vi "Funnel Edit.vi"() -> ()   [LabVIEW 2013]
uses:
  Global Variables.vi
panel:
  in  "Index":i32=8
  in  "Direction":u16(ring) items=["Forward", "Backward"]
  in  "Enabled":bool=TRUE
  in  "Voltage Schedule":u16(ring) items=["Constant", "Ramp", "Fn. Generator", "Formula"]
  in  "Apply to All":bool
  in  "Smooth Segments":dbl=12.0
  in  "Speed Schedule":u16(ring) items=["Constant", "Ramp", "Fn. Generator", "Formula"]
  in  "Speed (µm/s)":dbl=8.0 min=1e-09
  in  "Voltage (V)":dbl=8.0
  in  "Speed Settings":bool
  in  "Voltage Settings":bool
  in  "Bottom Segs.":dbl=0.1
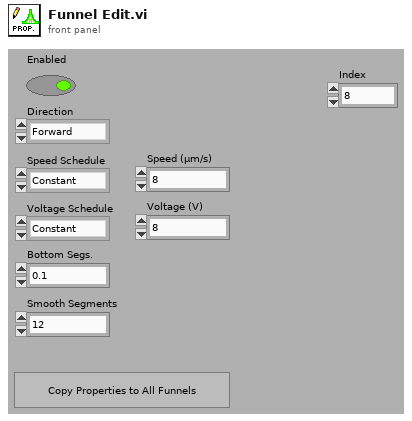
[diagram p1: front panel]
types:
  T1 = enum32{"invalid app kind", "Development System", "Run Time System", "Student Edition", "Embedded LabVIEW", "Evaluation", "Custom"}
  T2 = enum32{"Invalid", "Standard", "Closed", "Hidden", "Minimized", "Maximized"}
  T3 = cluster{"Enabled":bool, "Direction":u16, "Smooth Segments":dbl, "Bottom Segs.":dbl, "Speed (µm/s)":cluster{"Schedule":u16, "Value":dbl, "Start Value":dbl, "End Value":dbl, "Min Value":dbl, "Max Value":dbl, "Duty Cycle (%)":dbl, "Signal Type":u16, "Cycle Number":dbl, "Phase (degrees)":dbl}, "Voltage (V)":cluster{"Schedule":u16, "Value":dbl, "Start Value":dbl, "End Value":dbl, "Min Value":dbl, "Max Value":dbl, "Duty Cycle (%)":dbl, "Signal Type":u16, "Cycle Number":dbl, "Phase (degrees)":dbl}}[]
  T4 = cluster{"Enabled":bool, "Direction":u16, "Smooth Segments":dbl, "Bottom Segs.":dbl, "Speed (µm/s)":cluster{"Schedule":u16, "Value":dbl, "Start Value":dbl, "End Value":dbl, "Min Value":dbl, "Max Value":dbl, "Duty Cycle (%)":dbl, "Signal Type":u16, "Cycle Number":dbl, "Phase (degrees)":dbl}, "Voltage (V)":cluster{"Schedule":u16, "Value":dbl, "Start Value":dbl, "End Value":dbl, "Min Value":dbl, "Max Value":dbl, "Duty Cycle (%)":dbl, "Signal Type":u16, "Cycle Number":dbl, "Phase (degrees)":dbl}}
  T5 = cluster{"Schedule":u16, "Value":dbl, "Start Value":dbl, "End Value":dbl, "Min Value":dbl, "Max Value":dbl, "Duty Cycle (%)":dbl, "Signal Type":u16, "Cycle Number":dbl, "Phase (degrees)":dbl}
  T6 = cluster{"Schedule":u16, "Value":dbl, "Start Value":dbl, "End Value":dbl, "Min Value":dbl, "Max Value":dbl, "Duty Cycle (%)":dbl, "Speed Signal Type":u16, "Cycle Number":dbl, "Phase (degrees)":dbl}
  T7 = cluster{"Core":cluster{"Current VI Reference":refnum<vi>, "Close Panel on Exit?":bool}}
  T8 = cluster{"Current VI Reference":refnum<vi>, "Close Panel on Exit?":bool}
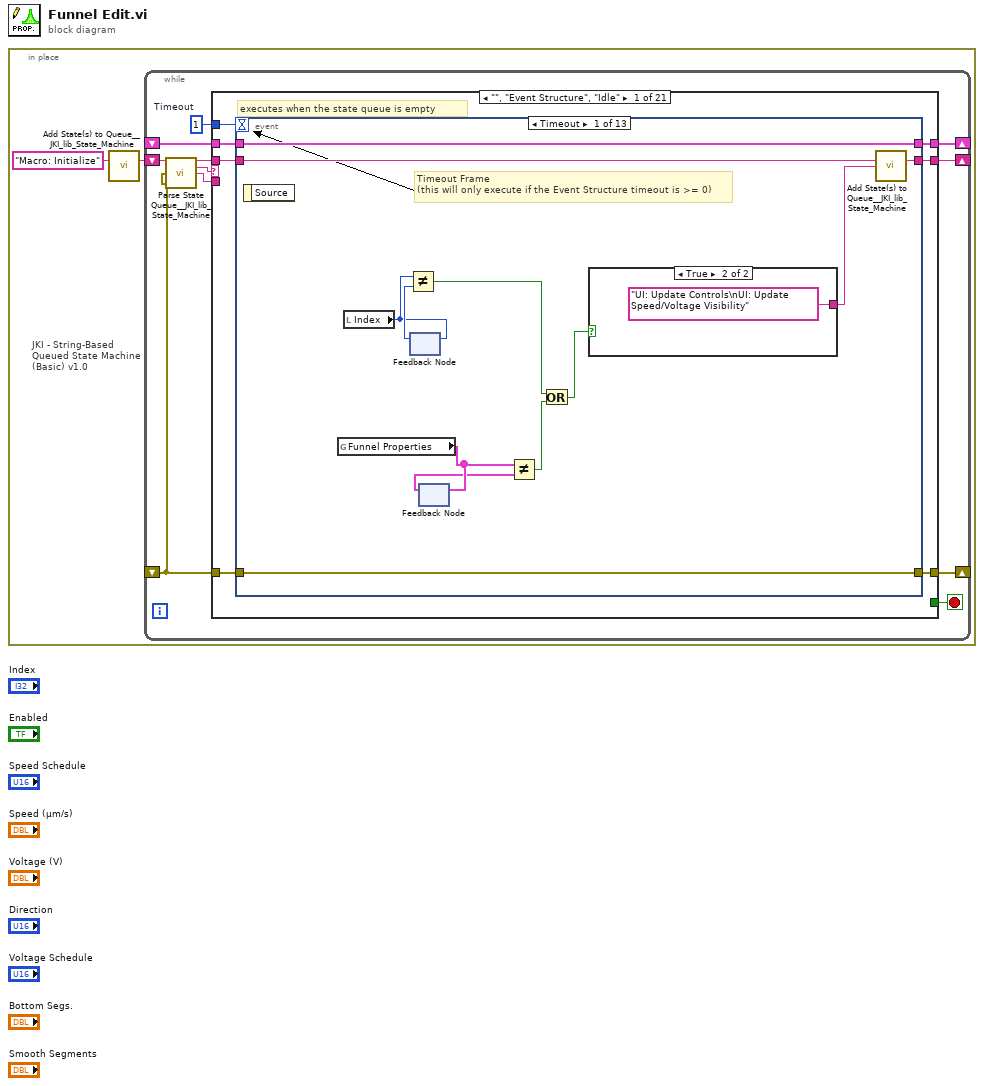
[diagram p0: block diagram]
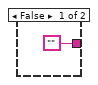
[diagram p2: hidden frame]
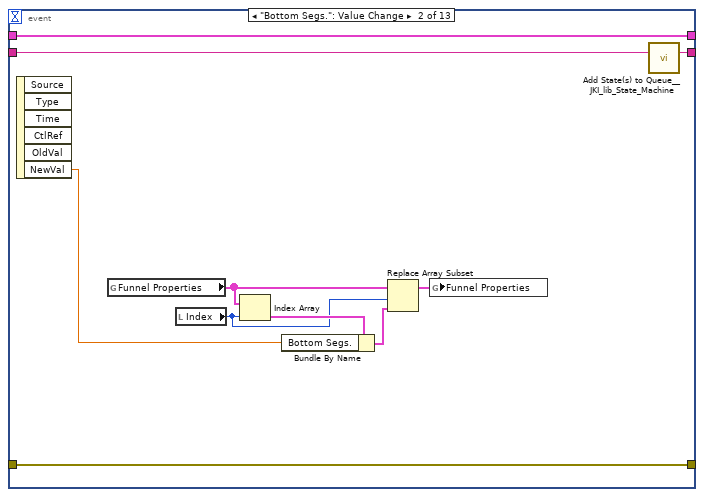
[diagram p3: hidden frame]
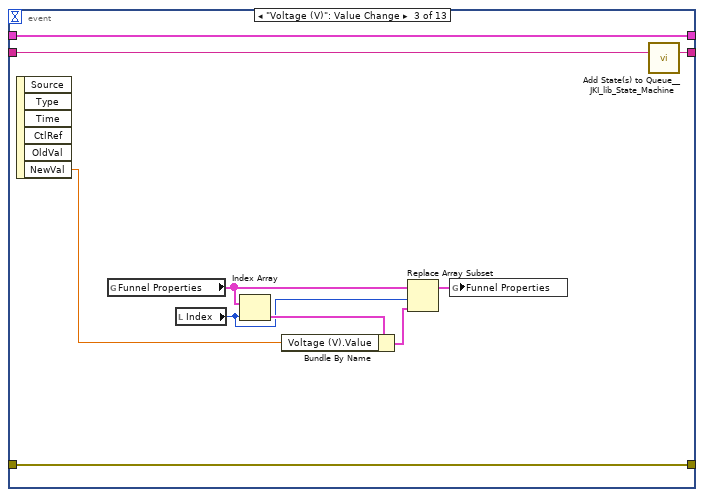
[diagram p4: hidden frame]
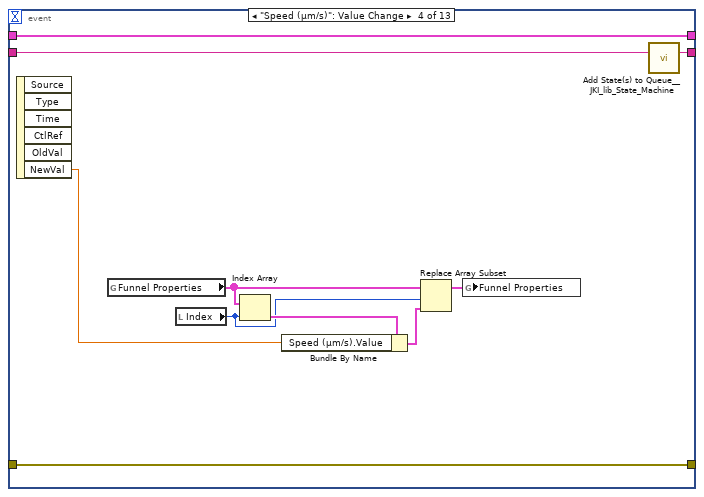
[diagram p5: hidden frame]
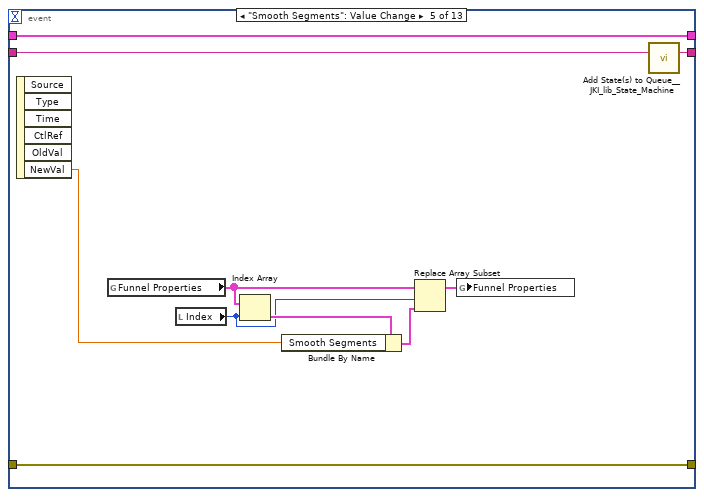
[diagram p6: hidden frame]
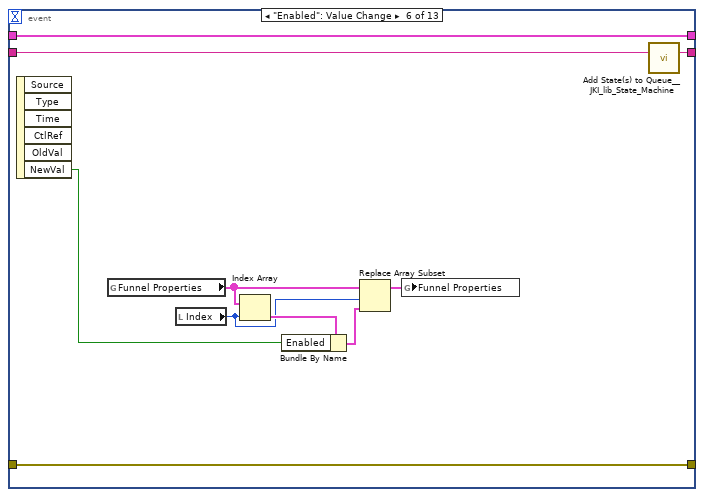
[diagram p7: hidden frame]
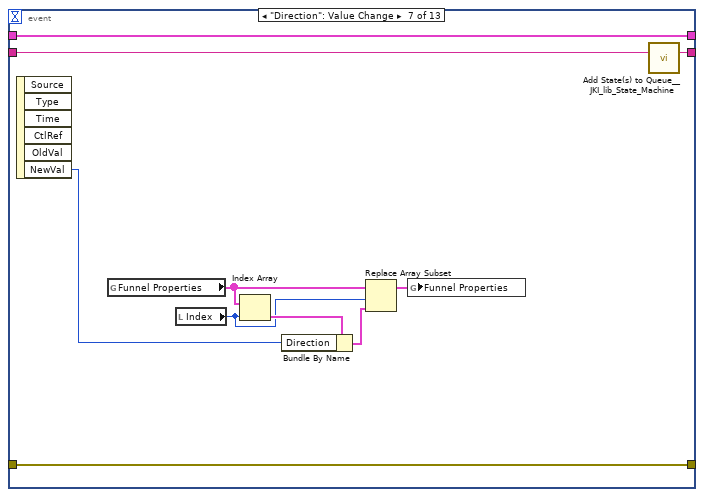
[diagram p8: hidden frame]
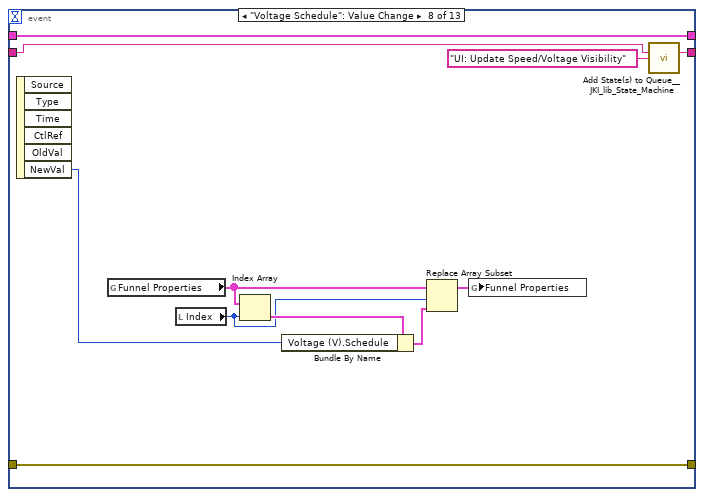
[diagram p9: hidden frame]
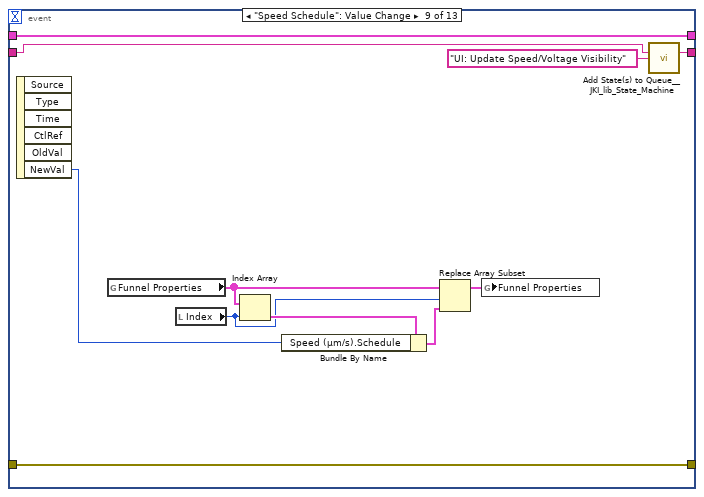
[diagram p10: hidden frame]
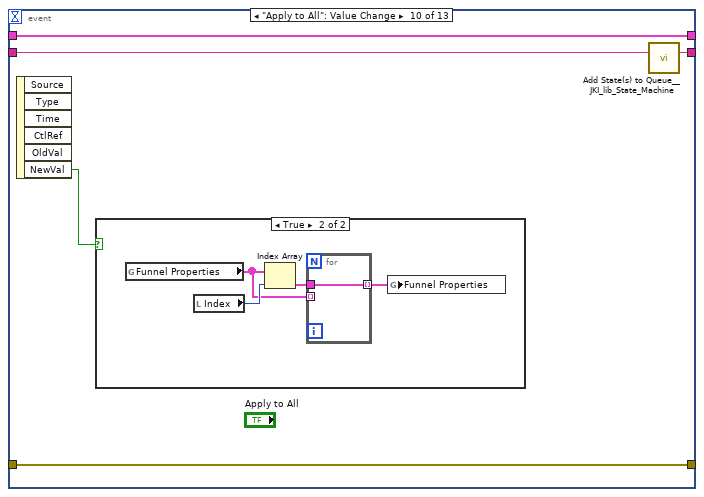
[diagram p11: hidden frame]
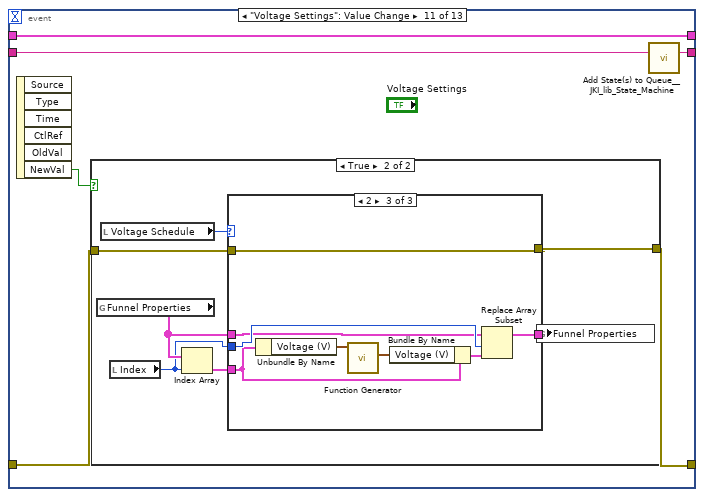
[diagram p13: hidden frame]
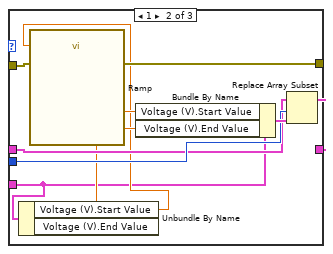
[diagram p16: hidden frame]
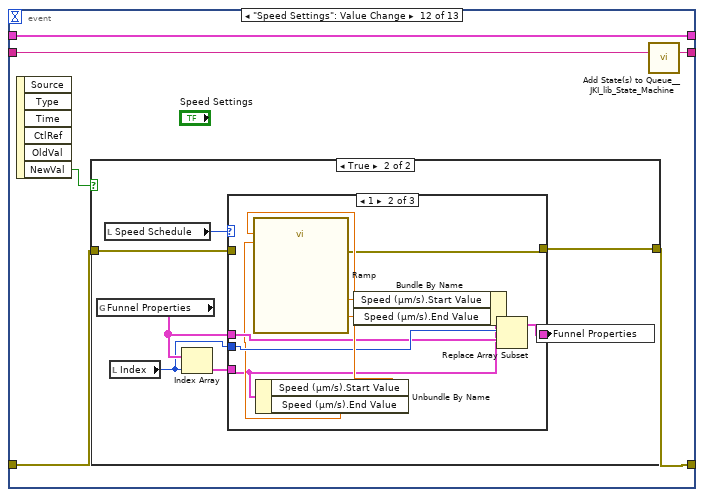
[diagram p17: hidden frame]
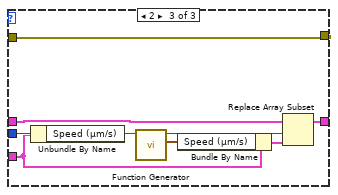
[diagram p20: hidden frame]
diagram:
  n1 = in-place {
    n2 = call <vilib>:"Add State(s) to Queue__JKI_lib_State_Machine.vi"("State(s) in (\"\")"="Macro: Initialize") -> ("States Out"=w2:string)  [unwired: 14 in]
    n3 = while "JKI - String-Based Queued State Machine (Basic) v1.0" {
      shift-right: [w6] -> _
      shift-left: _ -> [w5]
      shift-right: [w9] -> _
      shift-left: _ -> [w3]
      shift-right: [w8] -> _
      shift-left: w2 -> [w10]
      stop <- w7 stop-if-true
      w4 = 1  # Timeout
      n4 = call <vilib>:"Parse State Queue__JKI_lib_State_Machine.vi"("State Queue"=w10, "Error In (no error)"=w3) -> ("Remaining States"=w12:string, "Current State"=w13:string, "Arguments"=w11:string)  [unwired: 11 in]
      n5 = case shown="\"\", \"Event Structure\", \"Idle\"" w13 {
        selector: w13 -> [_ _ w206 _ _ _ _ _ _ _ _ _ _ _ _ _ _ _ _ _ _]
        tunnel: w12 -> [w20 w205 w210 w228 w234 w239 w243 w248 w254 w258 w262 w277 w283 w301 w312 w338 w343 w353 w357 w361 w365]
        tunnel: w11 -> [_ _ _ _ _ _ _ _ _ _ _ _ w278 _ w306 _ _ _ _ _ _]
        tunnel: w5 -> [w18 w202 w208 w224 w231 w237 w240 _ w252 w255 w260 w275 w281 w299 w308 w335 w340 w350 w354 w358 w362]
        tunnel: [w17 w203 w212 w225 errorcluster {"status"=FALSE, "code"=0, "source"=""} ("error out") w236 w241 w244 w250 w256 w259 w264 w279 w288 w309 w336 w341 w351 w355 w359 w363] -> w9
        tunnel: w3 -> [w16 w203 w211 w225 w230 w236 w241 w244 w249 w256 w259 w264 w280 w298 w310 w336 w341 w351 w355 w359 w363]
        tunnel: [w19 w204 w209 w227 w233 w238 w242 w247 w253 w257 w261 w276 w282 w300 w311 w337 w342 w352 w356 w360 w364] -> w8
        tunnel: [_ _ _ _ _ TRUE _ _ _ _ _ _ _ _ _ _ _ _ _ _ _] -> w7
        tunnel: [w15 w202 w208 w226 w231 w237 w240 w246 w252 w255 w260 w275 w281 w299 w308 w335 w340 w350 w354 w358 w362] -> w6
        tunnel: w4 -> [w14 _ _ _ _ _ _ _ _ _ _ _ _ _ _ _ _ _ _ _ _]
        frame "", "Event Structure", "Idle" {
          # "executes when the state queue is empty"
          n6 = event shown="[0] Timeout" {
            selector: _ -> [_ _ _ _ _ _ _ _ _ _ _ _ _]
            dyn-events: _ -> [_ _ _ _ _ _ _ _ _ _ _ _ _]
            timeout: w14 -> [_ _ _ _ _ _ _ _ _ _ _ _ _]
            tunnel: w20 -> [w32 w44 w54 w64 w74 w84 w94 w105 w116 w121 w132 w167 w201]
            tunnel: [w31 w43 w53 w63 w73 w83 w93 w104 w115 w120 w131 w166 w200] -> w19
            tunnel: w18 -> [w29 w42 w52 w62 w72 w82 w92 w103 w114 w119 w130 w165 w198]
            tunnel: [w30 w36 w46 w56 w66 w76 w86 w97 w108 w118 w128 w163 w199] -> w17
            tunnel: w16 -> [w30 w36 w46 w56 w66 w76 w86 w97 w108 w118 w129 w164 w199]
            tunnel: [w29 w42 w52 w62 w72 w82 w92 w103 w114 w119 w130 w165 w198] -> w15
            event Timeout {
              # "Timeout Frame\n(this will only execute if the Event Structure timeout is >= 0)"
              n7 = event-data() -> ()  [unwired: 1 in, 1 out]
              n8 = global read "Global Variables.vi" "Funnel Properties"() -> (w25:T3)
              n9 = local read "Index"() -> (w27:i32)
              n10 = feedback #1() -> (w28:i32)  [unwired: 1 in]
              n11 = Not Equal?(x=w27, y=w28) -> (x != y?=w23:bool)
              n12 = feedback-in #1(w27) -> ()
              n13 = feedback #2() -> (w24:T3)  [unwired: 1 in]
              n14 = feedback-in #2(w25) -> ()
              n15 = Not Equal?(x=w25, y=w24) -> (x != y?=w22:bool)
              n16 = Or(x=w23, y=w22) -> (x .or. y?=w21:bool)
              n17 = case shown="True" w21 {
                tunnel: ["" "UI: Update Controls\nUI: Update Speed/Voltage Visibility"] -> w26
                frame False {
                }
                frame True {
                }
              }
              n18 = call <vilib>:"Add State(s) to Queue__JKI_lib_State_Machine.vi"("State(s) in (\"\")"=w32, "State(s) at Back (\"\")"=w26) -> ("States Out"=w31:string)  [unwired: 13 in]
            }
            event "Bottom Segs.": Value Change {
              n19 = event-data() -> ("NewVal"=w40:dbl)  [unwired: 1 in, 5 out]
              n20 = global read "Global Variables.vi" "Funnel Properties"() -> (w38:T3)
              n21 = local read "Index"() -> (w35:i32)
              n22 = Index Array(array=w38, index=w35) -> (element=w41:T4)
              n23 = Bundle By Name(cluster=w41, "Bottom Segs."=w40) -> (w39:T4)
              n24 = Replace Array Subset(array=w38, new element=w39, index=w35) -> (w37:T3)
              n25 = global write "Global Variables.vi" "Funnel Properties"(w37) -> ()
              n26 = call <vilib>:"Add State(s) to Queue__JKI_lib_State_Machine.vi"("State(s) in (\"\")"=w44) -> ("States Out"=w43:string)  [unwired: 14 in]
            }
            event "Voltage (V)": Value Change {
              n27 = event-data() -> ("NewVal"=w50:dbl)  [unwired: 1 in, 5 out]
              n28 = global read "Global Variables.vi" "Funnel Properties"() -> (w48:T3)
              n29 = local read "Index"() -> (w45:i32)
              n30 = Index Array(array=w48, index=w45) -> (element=w51:T4)
              n31 = Bundle By Name(cluster=w51, "Voltage (V).Value"=w50) -> (w49:T4)
              n32 = Replace Array Subset(array=w48, new element=w49, index=w45) -> (w47:T3)
              n33 = global write "Global Variables.vi" "Funnel Properties"(w47) -> ()
              n34 = call <vilib>:"Add State(s) to Queue__JKI_lib_State_Machine.vi"("State(s) in (\"\")"=w54) -> ("States Out"=w53:string)  [unwired: 14 in]
            }
            event "Speed (µm/s)": Value Change {
              n35 = event-data() -> ("NewVal"=w60:dbl)  [unwired: 1 in, 5 out]
              n36 = global read "Global Variables.vi" "Funnel Properties"() -> (w58:T3)
              n37 = local read "Index"() -> (w55:i32)
              n38 = Index Array(array=w58, index=w55) -> (element=w61:T4)
              n39 = Bundle By Name(cluster=w61, "Speed (µm/s).Value"=w60) -> (w59:T4)
              n40 = Replace Array Subset(array=w58, new element=w59, index=w55) -> (w57:T3)
              n41 = global write "Global Variables.vi" "Funnel Properties"(w57) -> ()
              n42 = call <vilib>:"Add State(s) to Queue__JKI_lib_State_Machine.vi"("State(s) in (\"\")"=w64) -> ("States Out"=w63:string)  [unwired: 14 in]
            }
            event "Smooth Segments": Value Change {
              n43 = event-data() -> ("NewVal"=w70:dbl)  [unwired: 1 in, 5 out]
              n44 = global read "Global Variables.vi" "Funnel Properties"() -> (w68:T3)
              n45 = local read "Index"() -> (w65:i32)
              n46 = Index Array(array=w68, index=w65) -> (element=w71:T4)
              n47 = Bundle By Name(cluster=w71, "Smooth Segments"=w70) -> (w69:T4)
              n48 = Replace Array Subset(array=w68, new element=w69, index=w65) -> (w67:T3)
              n49 = global write "Global Variables.vi" "Funnel Properties"(w67) -> ()
              n50 = call <vilib>:"Add State(s) to Queue__JKI_lib_State_Machine.vi"("State(s) in (\"\")"=w74) -> ("States Out"=w73:string)  [unwired: 14 in]
            }
            event "Enabled": Value Change {
              n51 = event-data() -> ("NewVal"=w80:bool)  [unwired: 1 in, 5 out]
              n52 = global read "Global Variables.vi" "Funnel Properties"() -> (w78:T3)
              n53 = local read "Index"() -> (w75:i32)
              n54 = Index Array(array=w78, index=w75) -> (element=w81:T4)
              n55 = Bundle By Name(cluster=w81, "Enabled"=w80) -> (w79:T4)
              n56 = Replace Array Subset(array=w78, new element=w79, index=w75) -> (w77:T3)
              n57 = global write "Global Variables.vi" "Funnel Properties"(w77) -> ()
              n58 = call <vilib>:"Add State(s) to Queue__JKI_lib_State_Machine.vi"("State(s) in (\"\")"=w84) -> ("States Out"=w83:string)  [unwired: 14 in]
            }
            event "Direction": Value Change {
              n59 = event-data() -> ("NewVal"=w90:u16)  [unwired: 1 in, 5 out]
              n60 = global read "Global Variables.vi" "Funnel Properties"() -> (w88:T3)
              n61 = local read "Index"() -> (w85:i32)
              n62 = Index Array(array=w88, index=w85) -> (element=w91:T4)
              n63 = Bundle By Name(cluster=w91, "Direction"=w90) -> (w89:T4)
              n64 = Replace Array Subset(array=w88, new element=w89, index=w85) -> (w87:T3)
              n65 = global write "Global Variables.vi" "Funnel Properties"(w87) -> ()
              n66 = call <vilib>:"Add State(s) to Queue__JKI_lib_State_Machine.vi"("State(s) in (\"\")"=w94) -> ("States Out"=w93:string)  [unwired: 14 in]
            }
            event "Voltage Schedule": Value Change {
              n67 = event-data() -> ("NewVal"=w101:u16)  [unwired: 1 in, 5 out]
              n68 = global read "Global Variables.vi" "Funnel Properties"() -> (w99:T3)
              n69 = local read "Index"() -> (w95:i32)
              n70 = Index Array(array=w99, index=w95) -> (element=w102:T4)
              n71 = Bundle By Name(cluster=w102, "Voltage (V).Schedule"=w101) -> (w100:T4)
              n72 = Replace Array Subset(array=w99, new element=w100, index=w95) -> (w98:T3)
              n73 = global write "Global Variables.vi" "Funnel Properties"(w98) -> ()
              n74 = call <vilib>:"Add State(s) to Queue__JKI_lib_State_Machine.vi"("State(s) in (\"\")"=w105, "State(s) at Back (\"\")"="UI: Update Speed/Voltage Visibility" ("State(s) at Back (\"\")")) -> ("States Out"=w104:string)  [unwired: 13 in]
            }
            event "Speed Schedule": Value Change {
              n75 = event-data() -> ("NewVal"=w112:u16)  [unwired: 1 in, 5 out]
              n76 = global read "Global Variables.vi" "Funnel Properties"() -> (w110:T3)
              n77 = local read "Index"() -> (w106:i32)
              n78 = Index Array(array=w110, index=w106) -> (element=w113:T4)
              n79 = Bundle By Name(cluster=w113, "Speed (µm/s).Schedule"=w112) -> (w111:T4)
              n80 = Replace Array Subset(array=w110, new element=w111, index=w106) -> (w109:T3)
              n81 = global write "Global Variables.vi" "Funnel Properties"(w109) -> ()
              n82 = call <vilib>:"Add State(s) to Queue__JKI_lib_State_Machine.vi"("State(s) in (\"\")"=w116, "State(s) at Back (\"\")"="UI: Update Speed/Voltage Visibility" ("State(s) at Back (\"\")")) -> ("States Out"=w115:string)  [unwired: 13 in]
            }
            event "Apply to All": Value Change {
              n83 = event-data() -> ("NewVal"=w117:bool)  [unwired: 1 in, 5 out]
              n84 = case shown="True" w117 {
                frame False {
                }
                frame True {
                  n85 = global read "Global Variables.vi" "Funnel Properties"() -> (w122:T3)
                  n86 = local read "Index"() -> (w125:i32)
                  n87 = Index Array(array=w122, index=w125) -> (element=w124:T4)
                  n88 = for {
                    tunnel: w124 -> [w126]
                    tunnel: [w126] -> w123 mode=indexing
                    tunnel: w122 -> [_] mode=indexing
                  }
                  n89 = global write "Global Variables.vi" "Funnel Properties"(w123) -> ()
                }
              }
              n90 = call <vilib>:"Add State(s) to Queue__JKI_lib_State_Machine.vi"("State(s) in (\"\")"=w121) -> ("States Out"=w120:string)  [unwired: 14 in]
            }
            event "Voltage Settings": Value Change {
              n91 = event-data() -> ("NewVal"=w127:bool)  [unwired: 1 in, 5 out]
              n92 = case shown="True" w127 {
                tunnel: w129 -> [w133 w139]
                tunnel: [w133 w138] -> w128
                frame False {
                }
                frame True {
                  n93 = global read "Global Variables.vi" "Funnel Properties"() -> (w135:T3)
                  n94 = local read "Voltage Schedule"() -> (w140:u16)
                  n95 = local read "Index"() -> (w134:i32)
                  n96 = Index Array(array=w135, index=w134) -> (element=w136:T4)
                  n97 = case shown="2" w140 {
                    tunnel: w139 -> [w142 w153 w157]
                    tunnel: [w142 w146 w157] -> w138
                    tunnel: [w141 w147 w158] -> w137
                    tunnel: w136 -> [_ w143 w156]
                    tunnel: w135 -> [w141 w148 w159]
                    tunnel: w134 -> [_ w149 w160]
                    frame 0, Default {
                    }
                    frame 1 {
                      n98 = Unbundle By Name(w143) -> ("Voltage (V).Start Value"=w145:dbl, "Voltage (V).End Value"=w144:dbl)
                      n99 = call "Ramp.vi"("Start Value"=w145, "End Value"=w144, "error in (no error)"=w153) -> ("End Value"=w151:dbl, "Start Value"=w152:dbl, "error out"=w146:errorcluster)  [unwired: 13 in, 1 out]
                      n100 = Bundle By Name(cluster=w143, "Voltage (V).Start Value"=w152, "Voltage (V).End Value"=w151) -> (w150:T4)
                      n101 = Replace Array Subset(array=w148, new element=w150, index=w149) -> (w147:T3)
                    }
                    frame 2 {
                      n102 = Unbundle By Name(w156) -> ("Voltage (V)"=w154:T5)
                      n103 = call "Function Generator.vi"("Properties in"=w154) -> ("Properties out"=w155:T6)  [unwired: 9 in, 1 out]
                      n104 = Bundle By Name(cluster=w156, "Voltage (V)"=w155) -> (w161:T4)
                      n105 = Replace Array Subset(array=w159, new element=w161, index=w160) -> (w158:T3)
                    }
                  }
                  n106 = global write "Global Variables.vi" "Funnel Properties"(w137) -> ()
                }
              }
              n107 = call <vilib>:"Add State(s) to Queue__JKI_lib_State_Machine.vi"("State(s) in (\"\")"=w132) -> ("States Out"=w131:string)  [unwired: 14 in]
            }
            event "Speed Settings": Value Change {
              n108 = event-data() -> ("NewVal"=w162:bool)  [unwired: 1 in, 5 out]
              n109 = case shown="True" w162 {
                tunnel: w164 -> [w168 w174]
                tunnel: [w168 w173] -> w163
                frame False {
                }
                frame True {
                  n110 = global read "Global Variables.vi" "Funnel Properties"() -> (w170:T3)
                  n111 = local read "Speed Schedule"() -> (w175:u16)
                  n112 = local read "Index"() -> (w169:i32)
                  n113 = Index Array(array=w170, index=w169) -> (element=w171:T4)
                  n114 = case shown="1" w175 {
                    tunnel: w174 -> [w177 _ w191]
                    tunnel: [w177 w183 w191] -> w173
                    tunnel: [w176 w182 w192] -> w172
                    tunnel: w171 -> [_ w178 w190]
                    tunnel: w170 -> [w176 w180 w193]
                    tunnel: w169 -> [_ w181 w194]
                    frame 0, Default {
                    }
                    frame 1 {
                      n115 = Unbundle By Name(w178) -> ("Speed (µm/s).Start Value"=w184:dbl, "Speed (µm/s).End Value"=w179:dbl)
                      n116 = call "Ramp.vi"("Start Value"=w184, "End Value"=w179) -> ("End Value"=w186:dbl, "Start Value"=w187:dbl, "error out"=w183:errorcluster)  [unwired: 14 in, 1 out]
                      n117 = Bundle By Name(cluster=w178, "Speed (µm/s).Start Value"=w187, "Speed (µm/s).End Value"=w186) -> (w185:T4)
                      n118 = Replace Array Subset(array=w180, new element=w185, index=w181) -> (w182:T3)
                    }
                    frame 2 {
                      n119 = Unbundle By Name(w190) -> ("Speed (µm/s)"=w188:T5)
                      n120 = call "Function Generator.vi"("Properties in"=w188) -> ("Properties out"=w189:T6)  [unwired: 9 in, 1 out]
                      n121 = Bundle By Name(cluster=w190, "Speed (µm/s)"=w189) -> (w195:T4)
                      n122 = Replace Array Subset(array=w193, new element=w195, index=w194) -> (w192:T3)
                    }
                  }
                  n123 = global write "Global Variables.vi" "Funnel Properties"(w172) -> ()
                }
              }
              n124 = call <vilib>:"Add State(s) to Queue__JKI_lib_State_Machine.vi"("State(s) in (\"\")"=w167) -> ("States Out"=w166:string)  [unwired: 14 in]
            }
            event Panel Close? {
              # "Discard the event because we'll close the front panel ourselves in Macro: Exit"
              # "Close Panel button (pressed) Event\n(this executes Macro: Exit to terminate the VI)"
              n125 = event-data() -> ()  [unwired: 1 in, 1 out]
              n126 = event-data("Discard?"=TRUE) -> ()  [unwired: 1 in, 1 out]
              n127 = call <vilib>:"Add State(s) to Queue__JKI_lib_State_Machine.vi"("State(s) in Front (\"\")"="Macro: Exit", "State(s) in (\"\")"=w201) -> ("States Out"=w200:string)  [unwired: 13 in]
            }
          }
        }
        frame "---------- Core ----------" {
          # "Do not put any code in this frame.\n(it is a separator no-op)"
          n128 = call <vilib>:"Add State(s) to Queue__JKI_lib_State_Machine.vi"("State(s) in (\"\")"=w205) -> ("States Out"=w204:string)  [unwired: 14 in]
        }
        frame Default {
          w215 = 42 items=["No error", "Argument error", "Memory is full", "Out of zone", "End of file", "File already open", "Generic file I/O error", "File not found", "File permission error", "Disk is full", "Duplicate path", "Too many files open", "System feature not enabled", "Resource file not found", "Cannot add resource", "Resource not found", "Image not found", "Image memory error", "Pen does not exist", "Config type invalid", "Config token not found", "Config parse error", "Config memory error", "Bad external code format", "Bad external code offset", "External code not present", "Null window", "Destroy window error", "Null menu", "Print aborted", "Bad print record", "Print driver error", "Windows error during printing", "Memory error during printing", "Print dialog error", "Generic print error", "Invalid device refnum", "Device not found", "Device parameter error", "Device unit error", "Cannot open device", "Device call aborted", "Generic error", "Cancelled by user", "Object ID too low", "Object ID too high", "Object not in heap", "Unknown heap", "Unknown object (invalid DefProc)", "Unknown object (DefProc not in table)", "Message out of range", "Invalid (null) method", "Unknown message", "Manager call not supported", "Bad address", "Network operation in progress", "Network operation timed out", "Connection is busy", "Network attribute not supported", "Network error", "Address in use", "System out of memory", "Connection aborted", "Connection refused", "Not connected", "Already connected", "Connection closed", "Initialization error (interapplication manager)", "Bad occurrence", "Wait on unbound occurrence handler", "Occurrence queue overflow", "Datalog type conflict", "Unused", "Unrecognized type (interapplication manager)", "Memory corrupt", "Failed to make temporary DLL", "Old CIN version", "Drag socket not found", "Failed to load drop-object", "Failed to register OLE object", "Failed to release OLE object", "Format specifier type mismatch", "Unknown format specifier", "Too few format specifiers", "Too many format specifiers", "Scan failed", "Newer CIN version", "Error converting to variant", "Runtime menu error", "Password tampered", "Variant attribute not found", "Incompatible variant data type", "Event data is not available", "Event Store is not present", "Occurrence is not found", "Event Queue is not created", "Event info is not available", "Refnum passed is NULL", "Error retrieving Class GUID", "Error retrieving CoClass GUID", "Error retrieving TypeLib GUID.", "Bad built application magic bytes.", "Specific driver is different from the specific driver associated with the Logical Name.", "There is no session opened to the class driver.", "Max Error", "MAX - Error with config objects", "MAX - Error loading configuration", "MAX - Group not supported"]
          # "Current State"
          # "Do not delete, rename, or modify this frame.\n(this is used to capture unhandled states and typos)"
          # "Handle mistyped state name (developer tool)"
          n129 = Format Into String(format string="Software Exception: Unhandled State \"%s\"." ("message"), error in=w211, w206) -> (resulting string=w214:string, error out=w213:errorcluster)  [unwired: 1 in]
          n130 = call <vilib>:"Error Cluster From Error Code.vi"("show call chain? (False)"=TRUE, "error in (no error)"=w213, "error message (\"\")"=w214, "error code (0)"=w215) -> ("error out"=w212:errorcluster)  [unwired: 5 in]
          n131 = call <vilib>:"Add State(s) to Queue__JKI_lib_State_Machine.vi"("State(s) in (\"\")"=w210) -> ("States Out"=w209:string)  [unwired: 14 in]
        }
        frame "Initialize Core Data" {
          # "exe?"
          # "If panel starts closed or is an EXE, then close it when we exit"
          # "Do not delete, rename, or modify this frame.\n(this is used to determine panel behavior on exit)"
          n132 = property class="VI"() -> ("Front Panel.Open"=w222:bool)  [unwired: 2 in, 2 out]
          n133 = property class="App"() -> ("App.Kind"=w221:T1)  [unwired: 2 in, 2 out]
          n134 = control-ref of="Current VI Reference"() -> (w223:refnum<vi>)
          n135 = Not(x=w222) -> (.not. x?=w219:bool)
          n136 = Equal?(x=w221, y=T1."Run Time System" ("Application:Kind")) -> (x = y?=w218:bool)
          n137 = Or(x=w219, y=w218) -> (x .or. y?=w217:bool)
          n138 = Bundle By Name(cluster=w224, "Core.Current VI Reference"=w223, "Core.Close Panel on Exit?"=w217) -> (w226:T7)
          n139 = call <vilib>:"Add State(s) to Queue__JKI_lib_State_Machine.vi"("State(s) in (\"\")"=w228) -> ("States Out"=w227:string)  [unwired: 14 in]
        }
        frame "Error Handler" {
          # "Unhandled Error -- Display it"
          # "Handle any errors here.\nYou can also output any states to clean-up after errors occur"
          # "Clear error"
          n140 = call <vilib>:"General Error Handler.vi"("error in (no error)"=w230) -> ()  [unwired: 10 in, 5 out]
          n141 = call <vilib>:"Add State(s) to Queue__JKI_lib_State_Machine.vi"("State(s) in Front (\"\")"="/* Post Error States", "State(s) in (\"\")"=w234) -> ("States Out"=w233:string)  [unwired: 13 in]
        }
        frame "Exit" {
          # "Do not put any code in this frame.\n(No errors that occur here will be handled.)"
          n142 = call <vilib>:"Add State(s) to Queue__JKI_lib_State_Machine.vi"("State(s) in (\"\")"=w239) -> ("States Out"=w238:string)  [unwired: 14 in]
        }
        frame "---------- Data ----------" {
          # "Do not put any code in this frame.\n(It is a separator no-op. You can make a copy of this frame to create a new Data frame)"
          n143 = call <vilib>:"Add State(s) to Queue__JKI_lib_State_Machine.vi"("State(s) in (\"\")"=w243) -> ("States Out"=w242:string)  [unwired: 14 in]
        }
        frame "Data: Initialize" {
          w245 = T8 {"Current VI Reference"=refnum, "Close Panel on Exit?"=FALSE}  # Core
          # "Initialize the shift-register data, here.\n(data names are defined by what you wire into the bundle function)"
          n144 = Bundle("Core"=w245) -> (w246:T7)  [unwired: 1 in]
          n145 = call <vilib>:"Add State(s) to Queue__JKI_lib_State_Machine.vi"("State(s) in (\"\")"=w248) -> ("States Out"=w247:string)  [unwired: 14 in]
        }
        frame "Data: Cleanup" {
          # "Cleanup any data and references, here.\n(this is called automatically, by the Macro: Exit)"
          n146 = Unbundle By Name(w252) -> ("Core.Current VI Reference"=w251:refnum<vi>)
          n147 = Close Reference(reference=w251, error in (no error)=w249) -> (error out=w250:errorcluster)
          n148 = call <vilib>:"Add State(s) to Queue__JKI_lib_State_Machine.vi"("State(s) in (\"\")"=w254) -> ("States Out"=w253:string)  [unwired: 14 in]
        }
        frame "---------- UI ----------" {
          # "Do not put any code in this frame.\n(It is a separator no-op. You can make a copy of this frame to create a new UI frame)"
          n149 = call <vilib>:"Add State(s) to Queue__JKI_lib_State_Machine.vi"("State(s) in (\"\")"=w258) -> ("States Out"=w257:string)  [unwired: 14 in]
        }
        frame "UI: Initialize" {
          # "Initialize the User Interface, here.\n(this is called automatically, by the Macro: Init)"
          n150 = call <vilib>:"Add State(s) to Queue__JKI_lib_State_Machine.vi"("State(s) in (\"\")"=w262) -> ("States Out"=w261:string)  [unwired: 14 in]
        }
        frame "UI: Update Controls" {
          n151 = global read "Global Variables.vi" "Funnel Properties"() -> (w263:T3)
          n152 = local read "Index"() -> (w268:i32)
          n153 = Index Array(array=w263, index=w268) -> (element=w267:T4)
          n154 = Unbundle By Name(w267) -> ("Enabled"=w269:bool, "Direction"=w270:u16, "Smooth Segments"=w271:dbl, "Bottom Segs."=w272:dbl, "Speed (µm/s).Schedule"=w266:u16, "Speed (µm/s).Value"=w273:dbl, "Voltage (V).Schedule"=w265:u16, "Voltage (V).Value"=w274:dbl)
          n155 = local write "Enabled"(w269) -> ()
          n156 = local write "Direction"(w270) -> ()
          n157 = local write "Smooth Segments"(w271) -> ()
          n158 = local write "Bottom Segs."(w272) -> ()
          n159 = local write "Speed Schedule"(w266) -> ()
          n160 = local write "Speed (µm/s)"(w273) -> ()
          n161 = local write "Voltage Schedule"(w265) -> ()
          n162 = local write "Voltage (V)"(w274) -> ()
          n163 = call <vilib>:"Add State(s) to Queue__JKI_lib_State_Machine.vi"("State(s) in (\"\")"=w277) -> ("States Out"=w276:string)  [unwired: 14 in]
        }
        frame "UI: Cursor Set" {
          # "Argument"
          # "Set and Unset Cursor Busy.\n(Usage: \"UI: Cursor Set >> Busy|Idle\")"
          n164 = case shown="\"Idle\", Default" w278 {
            tunnel: w280 -> [w285 w287]
            tunnel: [w284 w286] -> w279
            frame "Idle", Default {
              n165 = call <vilib>:"Unset Busy.vi"("error in (no error)"=w285) -> ("error out"=w284:errorcluster)  [unwired: 10 in]
            }
            frame "Busy" {
              n166 = call <vilib>:"Set Busy.vi"("error in (no error)"=w287) -> ("error out"=w286:errorcluster)  [unwired: 9 in, 1 out]
            }
          }
          n167 = call <vilib>:"Add State(s) to Queue__JKI_lib_State_Machine.vi"("State(s) in (\"\")"=w283) -> ("States Out"=w282:string)  [unwired: 14 in]
        }
        frame "UI: Update Speed/Voltage Visibility" {
          n168 = local read "Voltage Schedule"() -> (w297:u16)
          n169 = case shown="0" w297 {
            tunnel: [TRUE FALSE] -> w293
            frame 0 {
            }
            frame 1, Default {
            }
          }
          n170 = local read "Speed Schedule"() -> (w296:u16)
          n171 = property on="Voltage (V)" class="DigNum (strict)"(error in=w298, "Visible"=w293) -> (error out=w294:errorcluster)  [unwired: 1 in, 1 out]
          n172 = case shown="0" w296 {
            tunnel: [TRUE FALSE] -> w289
            frame 0 {
            }
            frame 1, Default {
            }
          }
          n173 = Not(x=w293) -> (.not. x?=w292:bool)
          n174 = property on="Voltage Settings" class="Bool"(error in=w294, "Visible"=w292) -> (error out=w291:errorcluster)  [unwired: 1 in, 1 out]
          n175 = property on="Speed (µm/s)" class="DigNum (strict)"(error in=w291, "Visible"=w289) -> (error out=w290:errorcluster)  [unwired: 1 in, 1 out]
          n176 = Not(x=w289) -> (.not. x?=w295:bool)
          n177 = property on="Speed Settings" class="Bool"(error in=w290, "Visible"=w295) -> (error out=w288:errorcluster)  [unwired: 1 in, 1 out]
          n178 = call <vilib>:"Add State(s) to Queue__JKI_lib_State_Machine.vi"("State(s) in (\"\")"=w301) -> ("States Out"=w300:string)  [unwired: 14 in]
        }
        frame "UI: Front Panel State" {
          # "Argument"
          # "Set Front Panel Open or Closed\n(Usage: \"UI: Front Panel State >> Open|Close\")"
          n179 = Unbundle By Name(w308) -> ("Core.Current VI Reference"=w307:refnum<vi>)
          n180 = case shown="\"Open\", Default" w306 {
            tunnel: w310 -> [w316 w329]
            tunnel: [w318 w330] -> w309
            tunnel: w307 -> [w317 w327]
            frame "Open", Default {
              n181 = property class="VI"(reference=w317, error in=w316) -> (reference out=w314:refnum<vi>, error out=w315:errorcluster, "Front Panel.Open"=w313:bool)
              n182 = case shown="False" w313 {
                tunnel: [w321 w324] -> w318
                tunnel: w315 -> [w320 w324]
                tunnel: w314 -> [w319 _]
                frame False {
                  n183 = invoke class="VI" method="FP.Open"(reference=w319, error in=w320, "Activate"=TRUE, "State"=T2."Standard") -> (error out=w321:errorcluster)  [unwired: 1 in, 4 out]
                }
                frame True {
                }
              }
            }
            frame "Close" {
              n184 = property class="VI"(reference=w327, error in=w329) -> (reference out=w326:refnum<vi>, error out=w328:errorcluster, "Front Panel.Open"=w325:bool)
              n185 = case shown="True" w325 {
                tunnel: [w331 w334] -> w330
                tunnel: w328 -> [w331 w333]
                tunnel: w326 -> [_ w332]
                frame False {
                }
                frame True {
                  n186 = invoke class="VI" method="FP.Close"(reference=w332, error in=w333) -> (error out=w334:errorcluster)  [unwired: 1 in, 2 out]
                }
              }
            }
          }
          n187 = call <vilib>:"Add State(s) to Queue__JKI_lib_State_Machine.vi"("State(s) in (\"\")"=w312) -> ("States Out"=w311:string)  [unwired: 14 in]
        }
        frame "---------- Macro ----------" {
          # "Do not put any code in this frame.\n(It is a separator no-op. You can make a copy of this frame to create a new Macro frame)"
          n188 = call <vilib>:"Add State(s) to Queue__JKI_lib_State_Machine.vi"("State(s) in (\"\")"=w338) -> ("States Out"=w337:string)  [unwired: 14 in]
        }
        frame "Macro: Initialize" {
          w339 = "Data: Initialize\nInitialize Core Data\nUI: Initialize\nUI: Update Controls\nUI: Update Speed/Voltage Visibility\nUI: Front Panel State >> Close"  # Data: Initialize Initialize Core Data UI: Initialize UI: Update Controls UI: Update Speed/Voltage Visibility UI: Front Panel State >> Close
          # "Initialization Macro\n(This is called once, when the VI starts)"
          n189 = call <vilib>:"Add State(s) to Queue__JKI_lib_State_Machine.vi"("State(s) in Front (\"\")"=w339, "State(s) in (\"\")"=w343) -> ("States Out"=w342:string)  [unwired: 13 in]
        }
        frame "Macro: Exit" {
          # "Exit Macro\n(This is called once, when the VI exits)"
          n190 = Unbundle By Name(w350) -> ("Core.Close Panel on Exit?"=w349:bool)
          n191 = Select(t="UI: Front Panel State >> Close", s=w349, f="") -> (s? t:f=w346:string)
          n192 = call <vilib>:"Add State(s) to Queue__JKI_lib_State_Machine.vi"("State(s) in (\"\")"=w346, "State(s) at Back (\"\")"="Data: Cleanup\nExit") -> ("States Out"=w344:string)  [unwired: 13 in]
          n193 = call <vilib>:"Add State(s) to Queue__JKI_lib_State_Machine.vi"("State(s) in Front (\"\")"=w344, "State(s) in (\"\")"=w353) -> ("States Out"=w352:string)  [unwired: 13 in]
        }
        frame "---------- New Category ----------" {
          # "Template Separator\n(You can make a copy of, or modify, this frame)"
          n194 = call <vilib>:"Add State(s) to Queue__JKI_lib_State_Machine.vi"("State(s) in (\"\")"=w357) -> ("States Out"=w356:string)  [unwired: 14 in]
        }
        frame "New Category: 1" {
          # "Your code here.\n(You can make a copy of, or modify, this frame)"
          n195 = call <vilib>:"Add State(s) to Queue__JKI_lib_State_Machine.vi"("State(s) in (\"\")"=w361) -> ("States Out"=w360:string)  [unwired: 14 in]
        }
        frame "New Category: 2" {
          # "Your code here.\n(You can make a copy of, or modify, this frame)"
          n196 = call <vilib>:"Add State(s) to Queue__JKI_lib_State_Machine.vi"("State(s) in (\"\")"=w365) -> ("States Out"=w364:string)  [unwired: 14 in]
        }
      }
    }
  }
